vi "scaleFactor.get.vi"(8 "error in (no error)":errorcluster, 11 "scaleFactor in":refnum<class "scaleFactor.lvclass">) -> (0 "error out":errorcluster, 2 "scaleFactor":dbl, 3 "scaleFactor out":refnum<class "scaleFactor.lvclass">)   [LabVIEW 2020, in "nominal types.lvlib" / "timestampManifest.lvlib" / "scaleFactor.lvclass"]
uses:
  scaleFactor.lvclass
  scaleFactor.lvclass/scaleFactor.ctl
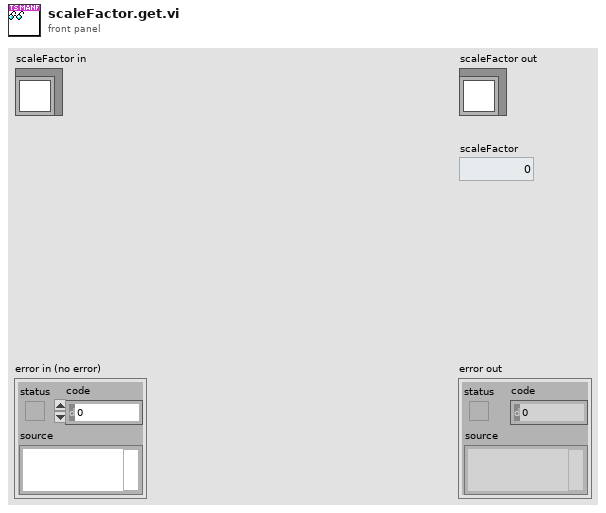
[diagram p1: front panel]
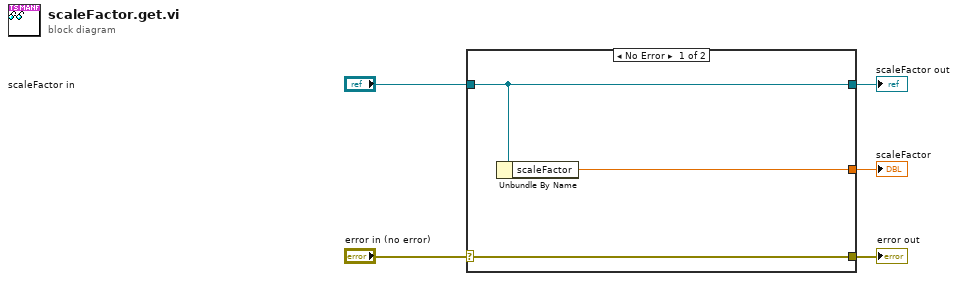
[diagram p0: block diagram]
diagram:
  n1 = case shown="No Error" "error in (no error)" {
    selector: "error in (no error)" -> [w8 w9]
    tunnel: [w8 w9] -> w4
    tunnel: [w7 w10] -> w2
    tunnel: "scaleFactor in" -> [w7 w10]
    tunnel: [w6 _] -> w1
    frame No Error {
      n2 = Unbundle By Name(w7) -> ("scaleFactor"=w6:dbl)
    }
    frame Error {
    }
  }
  "error out" <- w4
  "scaleFactor out" <- w2
  "scaleFactor" <- w1
